vi "Get DataBindings.vi"(8 "error in":errorcluster caption="entrée d'erreur (pas d'erreur)", 11 "Experiment.lvclass":refnum<class "Experiment.lvclass">) -> (0 "error out":errorcluster caption="sortie d'erreur", 3 "Experiment.lvclass out":refnum<class "Experiment.lvclass">)   [LabVIEW 2019, in "Experiment.lvclass"]
uses:
  Experiment.lvclass
  Experiment.lvclass/Experiment.ctl
  DevicesClass/BaseDevice/ClassQueueMess.ctl
  DevicesClass/BaseDevice/BaseDevice.lvclass
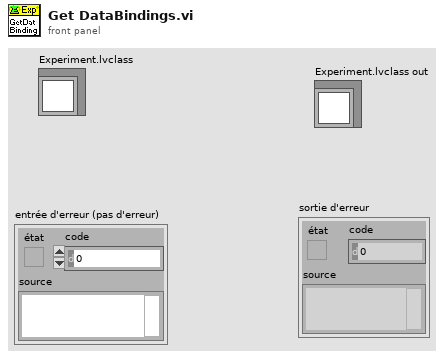
[diagram p1: front panel]
types:
  T1 = typedef "ClassQueueMess.ctl" = u16
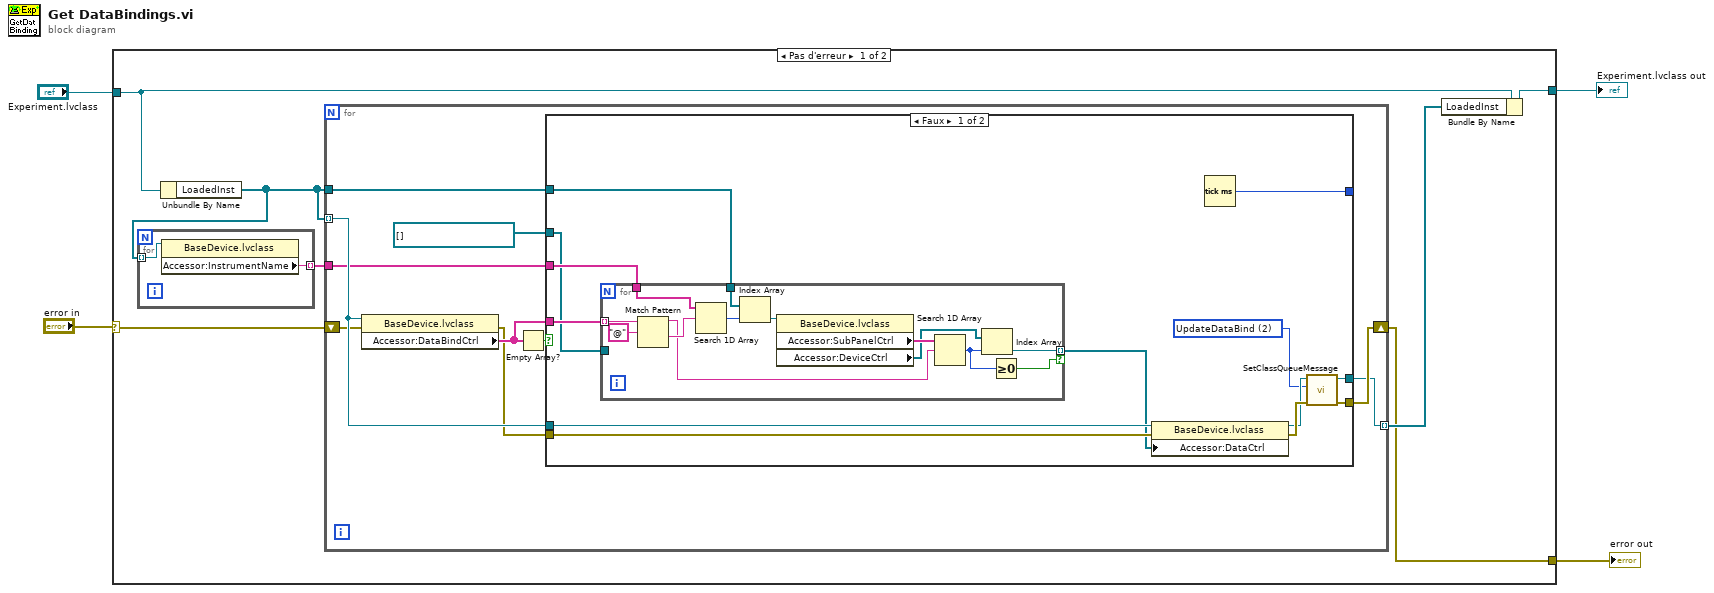
[diagram p0: block diagram]
diagram:
  n1 = case shown="Pas d'erreur" "error in" {
    selector: "error in" -> [w10 w53]
    tunnel: [w7 w52] -> w4
    tunnel: "Experiment.lvclass" -> [w11 w52]
    tunnel: [w5 w53] -> w1
    frame No Error {
      n2 = Unbundle By Name(w11) -> ("LoadedInst"=w9:refnum<class "BaseDevice.lvclass">[])
      n3 = for {
        tunnel: w9 -> [w13] mode=indexing
        tunnel: [w12] -> w8 mode=indexing
        n4 = property class="BaseDevice.lvclass"(reference=w13) -> ("Accessor:InstrumentName"=w12:string)  [unwired: 1 in, 2 out]
      }
      n5 = for {
        tunnel: w9 -> [w20] mode=indexing
        tunnel: w9 -> [w21]
        tunnel: [w14] -> w6 mode=indexing
        shift-right: [w15] -> w5
        shift-left: w10 -> [w18]
        tunnel: w8 -> [w17]
        n6 = property class="BaseDevice.lvclass"(reference=w20, error in=w18) -> (error out=w19:errorcluster, "Accessor:DataBindCtrl"=w22:string[])  [unwired: 1 out]
        n7 = Empty Array?(array=w22) -> (empty?=w23:bool)
        n8 = case shown="Faux" w23 {
          tunnel: w22 -> [w36 _]
          tunnel: w21 -> [w35 _]
          tunnel: w20 -> [w31 w51]
          tunnel: w19 -> [w32 w50]
          tunnel: w17 -> [w34 _]
          tunnel: refnum<vi>[] [] -> [w33 _]
          tunnel: [w29 _] -> _
          tunnel: [w26 w50] -> w15
          tunnel: [w25 w51] -> w14
          frame False {
            w24 = T1 2 items=["UpdateClassData", "UpdateMainClass", " UpdateDataBind "] ("Menu déroulant")
            n9 = for {
              tunnel: w36 -> [w48] mode=indexing
              tunnel: w34 -> [w47]
              tunnel: w35 -> [w45]
              tunnel: w33 -> [_]
              tunnel: [w38] -> w30 mode=indexing if=w37
              n10 = Match Pattern(string=w48, regular expression="@" ("expression régulière")) -> (before substring=w41:string, after substring=w46:string)  [unwired: 1 in, 2 out]
              n11 = Search 1D Array(1D array=w47, element=w46) -> (index of element=w44:i32)  [unwired: 1 in]
              n12 = Index Array(array=w45, index=w44) -> (element=w43:refnum<class "BaseDevice.lvclass">)
              n13 = property class="BaseDevice.lvclass"(reference=w43) -> ("Accessor:SubPanelCtrl"=w42:string[], "Accessor:DeviceCtrl"=w40:refnum<vi>[])  [unwired: 1 in, 2 out]
              n14 = Search 1D Array(1D array=w42, element=w41) -> (index of element=w39:i32)  [unwired: 1 in]
              n15 = Index Array(array=w40, index=w39) -> (element=w38:refnum<vi>)
              n16 = Greater Or Equal To 0?(x=w39) -> (x >= 0?=w37:bool)
            }
            n17 = property class="BaseDevice.lvclass"(reference=w31, error in=w32, "Accessor:DataCtrl"=w30) -> (reference out=w27:refnum<class "BaseDevice.lvclass">, error out=w28:errorcluster)
            n18 = Tick Count (ms)() -> (millisecond timer value=w29:u32)
            n19 = call-dynamic "SetClassQueueMessage.vi"("ErrorIn(No Error)"=w28, "Menu déroulant"=w24, "BaseDevice.lvclass"=w27) -> ("sortie d'erreur"=w26:errorcluster, "BaseDevice.lvclass Out"=w25:refnum<class "BaseDevice.lvclass">)  [unwired: 7 in]
          }
          frame True {
          }
        }
      }
      n20 = Bundle By Name(cluster=w11, "LoadedInst"=w6) -> (w7:refnum<class "Experiment.lvclass">)
    }
    frame Error {
    }
  }
  "Experiment.lvclass out" <- w4
  "error out" <- w1
